vi "io_translate.vi"(7 "mode":T1, 8 "error in (no error)":errorcluster, 10 "vector":dbl[](array[numeric])=[0.0, 0.0, 0.0], 11 "points in":dbl[][](array[numeric])) -> (0 "error out":errorcluster, 3 "points out":dbl[][](array[numeric]))   [LabVIEW 2010, in "PointCollection.lvclass"]
uses:
  PointCollection.lvclass
  mode_enum.ctl
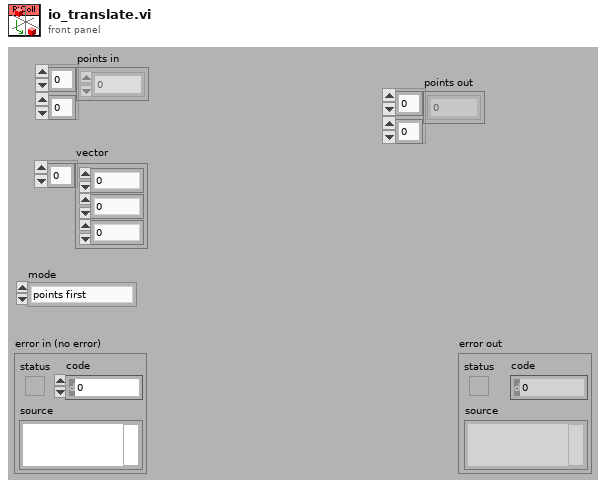
[diagram p1: front panel]
types:
  T1 = typedef "PointCollection.lvclass/mode_enum.ctl" = enum16{"points first", "dimensions first"}
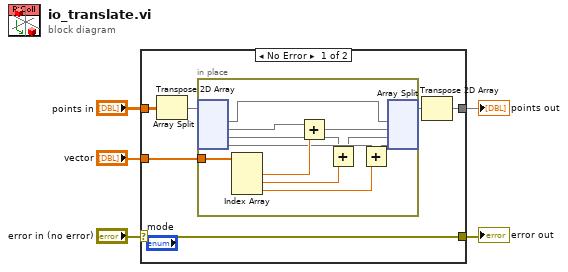
[diagram p0: block diagram]
diagram:
  n1 = case shown="No Error" "error in (no error)" {
    selector: "error in (no error)" -> [w11 w24]
    tunnel: [w11 w24] -> w4
    tunnel: "vector" -> [w10 _]
    tunnel: "points in" -> [w9 w23]
    tunnel: [w6 w23] -> w1
    frame No Error {
      n2 = Transpose 2D Array(2D array=w9) -> (transposed array=w8:dbl[][])
      n3 = in-place {
        in-place-border: w10 -> [w22]
        n4 = in-place-split #1(w8) -> (w12:dbl[][], w14:dbl[][], w16:dbl[][], w18:dbl[][])  [unwired: 3 in]
        n5 = Index Array(array=w22) -> (element #1=w21:dbl, element #2=w20:dbl, element #3=w19:dbl)  [unwired: 3 in]
        n6 = Add(x=w14, y=w21) -> (x+y=w13:dbl[][])
        n7 = Add(x=w16, y=w20) -> (x+y=w15:dbl[][])
        n8 = Add(x=w18, y=w19) -> (x+y=w17:dbl[][])
        n9 = in-place-split #1(w12, w13, w15, w17) -> (w7:dbl[][])  [unwired: 3 out]
      }
      n10 = Transpose 2D Array(2D array=w7) -> (transposed array=w6:dbl[][])
    }
    frame Error {
    }
  }
  "error out" <- w4
  "points out" <- w1
